vi "74LS138实现任意组合逻辑.vi"() -> ()   [LabVIEW 2018]
panel:
  in  "结束":bool
  out "灯":bool
  in  "开关C":bool
  in  "开关B":bool
  in  "开关A":bool
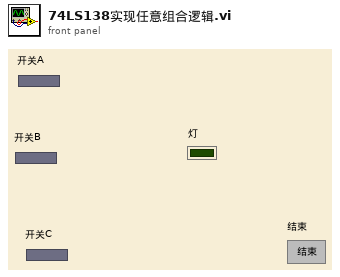
[diagram p1: front panel]
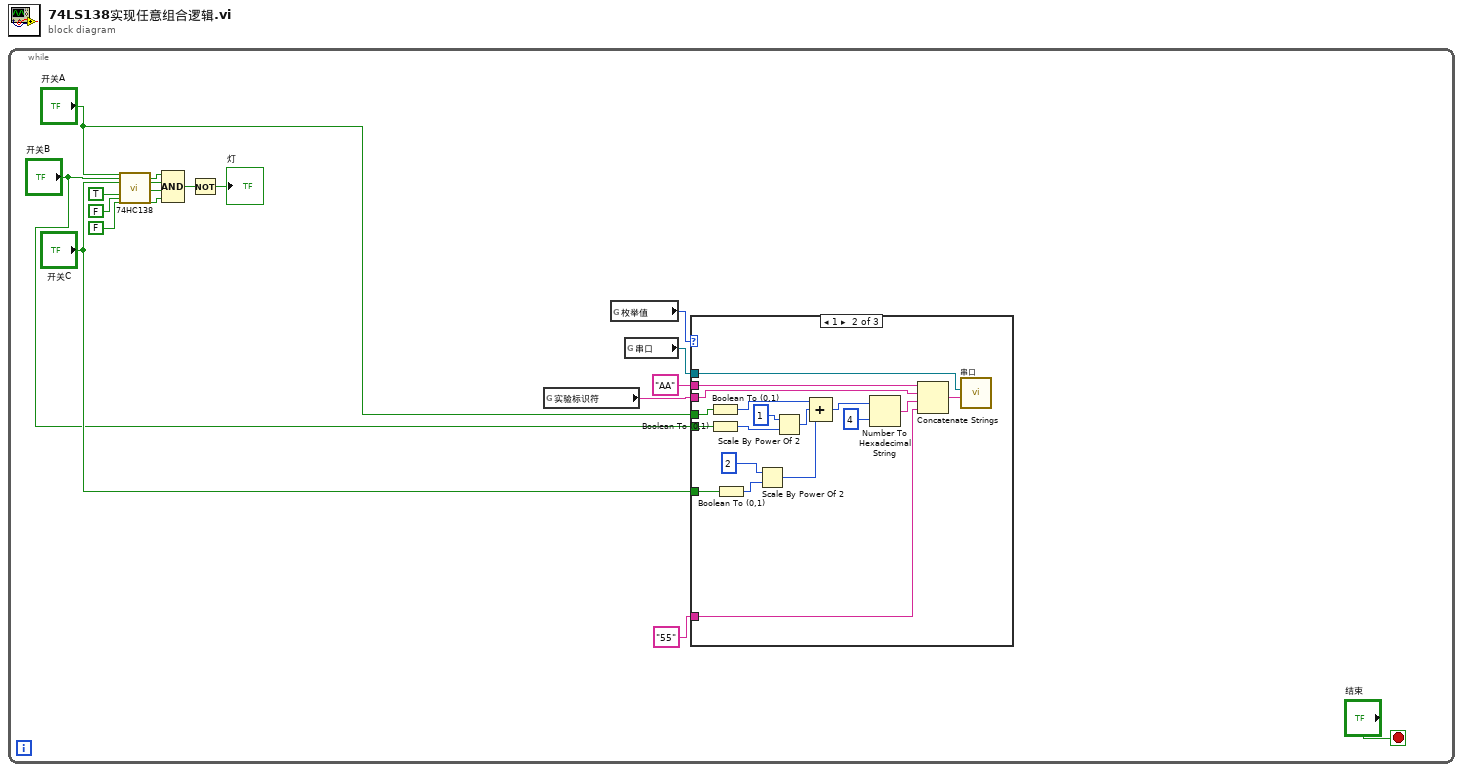
[diagram p0: block diagram]
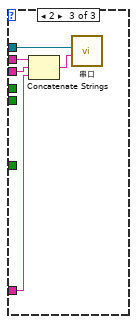
[diagram p3: hidden frame]
diagram:
  n1 = while {
    stop <- "结束" stop-if-true
    n2 = call "74HC138.vi"("A0"="开关A", "A1"="开关B", "A2"="开关C", "S1"=TRUE, "S2`"=FALSE, "S3`"=FALSE) -> ("Y1`"=w14:bool, "Y2`"=w13:bool, "Y4`"=w12:bool, "Y7`"=w11:bool)  [unwired: 14 in, 4 out]
    n3 = Compound Arithmetic op=AND ("复合运算")(w14, w13, w12, w11) -> (w15:bool)
    n4 = Not(x=w15) -> (.not. x?=→"灯":bool)
    n5 = global read "全局变量.vi" "实验标识符"() -> (w6:string)
    n6 = global read "全局变量.vi" "枚举值"() -> (w8:i8)
    n7 = global read "全局变量.vi" "串口"() -> (w7:refnum<visa-resource-name>)
    n8 = case shown="1" w8 {
      tunnel: w7 -> [_ w31 w39]
      tunnel: w6 -> [_ w30 w40]
      tunnel: "55" -> [_ w29 w37]
      tunnel: "AA" -> [_ w28 w38]
      tunnel: "开关A" -> [_ w21 _]
      tunnel: "开关C" -> [_ w20 _]
      tunnel: "开关B" -> [_ w19 _]
      frame 0, Default {
      }
      frame 1 {
        n9 = Boolean To (0,1)(Boolean=w21) -> (0, 1=w35:i16)
        n10 = Boolean To (0,1)(Boolean=w19) -> (0, 1=w33:i16)
        n11 = Boolean To (0,1)(Boolean=w20) -> (0, 1=w23:i16)
        n12 = Scale By Power Of 2(n=2, x=w23) -> (x*2^n=w24:i16)
        n13 = Scale By Power Of 2(n=1, x=w33) -> (x*2^n=w34:i16)
        n14 = Compound Arithmetic op=ADD ("复合运算")(w35, w34, w24) -> (w27:i16)
        n15 = Number To Hexadecimal String(1:4, 2:w27) -> (0:w25:string)
        n16 = Concatenate Strings(w28, w30, w25, w29) -> (w36:string)
        n17 = call "串口.vi"("字符串"=w36, "VISA resource name"=w31) -> ()  [unwired: 10 in]
      }
      frame 2 {
        n18 = Concatenate Strings(w38, w40, w37) -> (w41:string)
        n19 = call "串口.vi"("字符串"=w41, "VISA resource name"=w39) -> ()  [unwired: 10 in]
      }
    }
  }
